vi "norm_vec.vi"(4 "vector":dbl[](array[numeric])) -> (0 "magnitude":dbl, 1 "normalized vector":dbl[](array[numeric]))   [LabVIEW 2013]
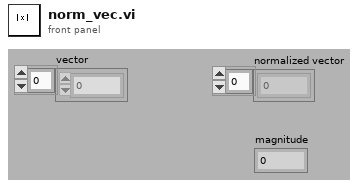
[diagram p1: front panel]
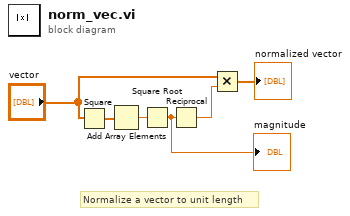
[diagram p0: block diagram]
diagram:
  # "Normalize a vector to unit length"
  n1 = Square(x="vector") -> (x^2=w6:dbl[])
  n2 = Add Array Elements(numeric array=w6) -> (sum=w5:dbl)
  n3 = Square Root(x=w5) -> (sqrt(x)=w1:dbl)
  "magnitude" <- w1
  n4 = Reciprocal(x=w1) -> (1/x=w4:dbl)
  n5 = Multiply ("Multiply.vi")(x="vector", y=w4) -> (x*y=→"normalized vector":dbl[])
